vi "EXA_RCL_STATE.vi"(6 "FileName":string, 8 "error in":errorcluster {"code" format="%.0x"}, 11 "Session In":refnum<visa-resource-name>="TCPIP0::K-N90X0A-00005.local::hislip0::INSTR") -> (0 "error out":errorcluster {"code" format="%.0x"}, 3 "Session Out":refnum<visa-resource-name>)   [LabVIEW 2018]
panel:
  in  "Timeout":u32=3000
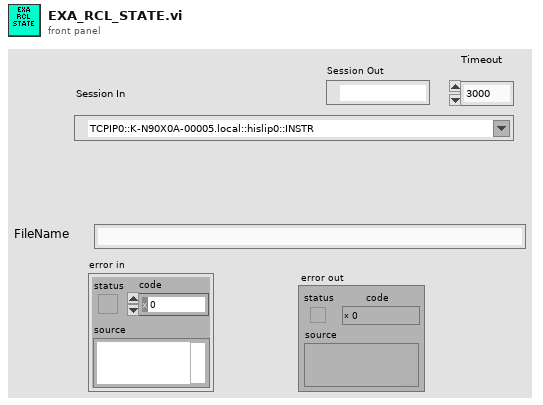
[diagram p1: front panel]
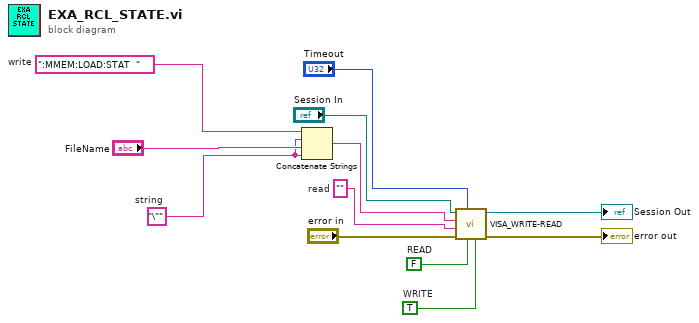
[diagram p0: block diagram]
diagram:
  w3 = TRUE  # WRITE
  w4 = FALSE  # READ
  w1 = "\""  # string
  w9 = ""  # read
  w2 = ":MMEM:LOAD:STAT  "  # write
  n1 = Concatenate Strings(w2, w1, "FileName", w1) -> (w10:string)
  n2 = call "VISA_WRITE-READ.vi"("WRITE"=w3, "READ"=w4, "Timeout"="Timeout", "error in"="error in", "Rcmd"=w9, "Wcmd"=w10, "Session In"="Session In") -> ("error out"=→"error out":errorcluster, "Session Out"=→"Session Out":refnum<visa-resource-name>)  [unwired: 2 in, 1 out]
